vi "waitForArduino.vi"(11 "VISA Refnum in":refnum<visa-resource-name>) -> (2 "Boolean":bool, 3 "VISA Refnum out":refnum<visa-resource-name>)   [LabVIEW 2021]
panel:
  out "read buffer":string
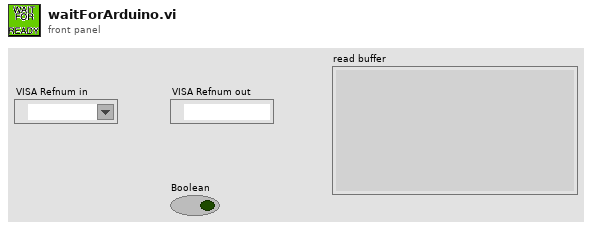
[diagram p1: front panel]
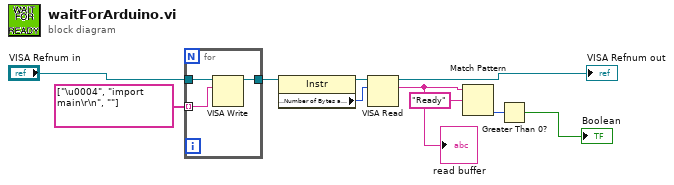
[diagram p0: block diagram]
diagram:
  n1 = for {
    tunnel: string[] ["\u0004", "import main\r\n", ""] -> [w12] mode=indexing
    tunnel: "VISA Refnum in" -> [w13]
    tunnel: [w11] -> w2
    n2 = VISA Write(VISA resource name=w13, write buffer=w12) -> (VISA resource name out=w11:refnum<visa-resource-name>)  [unwired: 1 in, 2 out]
  }
  n3 = property class="Instr"(reference=w2) -> (reference out=w5:refnum<visa-resource-name>, "Serial Settings:Number of Bytes at Serial Port"=w4:u32)  [unwired: 1 in, 1 out]
  n4 = VISA Read(VISA resource name=w5, byte count=w4) -> (VISA resource name out=→"VISA Refnum out":refnum<visa-resource-name>, read buffer=w6:string)  [unwired: 1 in, 2 out]
  "read buffer" <- w6
  n5 = Match Pattern(string=w6, regular expression="Ready") -> (offset past match=w8:i32)  [unwired: 1 in, 3 out]
  n6 = Greater Than 0?(x=w8) -> (x > 0?=→"Boolean":bool)
